vi "Write Idle read.vi"(8 "error in (no error)":errorcluster, 10 "Idle read?":bool, 11 "BaseDriver in":refnum<class "BaseDriver.lvclass">) -> (0 "error out":errorcluster, 3 "BaseDriver out":refnum<class "BaseDriver.lvclass">)   [LabVIEW 2013, in "BaseDriver.lvclass"]
doc: "Determines the drivers behaviour when there is no data to read and no data to send to the remote destination. If Idle Read is true, the driver will wait for data from the remote destination to become available, otherwise it will wait for data from the calling application to become available. It will have slightly faster response time to incoming data from the source it is waiting on.\n\nYour driver should wait for the party that most often initiates communication."
uses:
  BaseDriver.lvclass
  BaseDriver.lvclass/BaseDriver.ctl
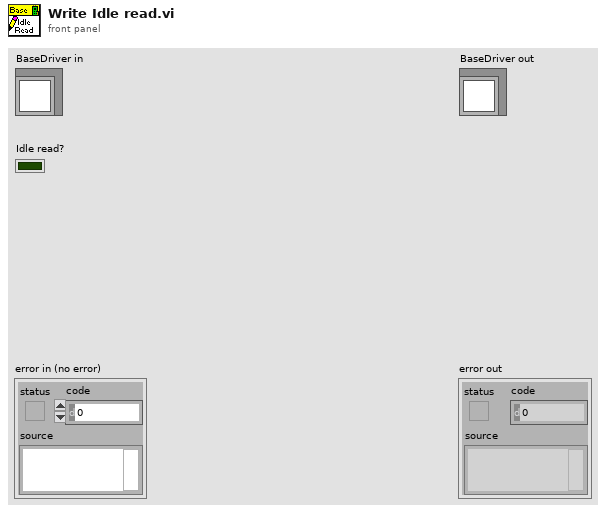
[diagram p1: front panel]
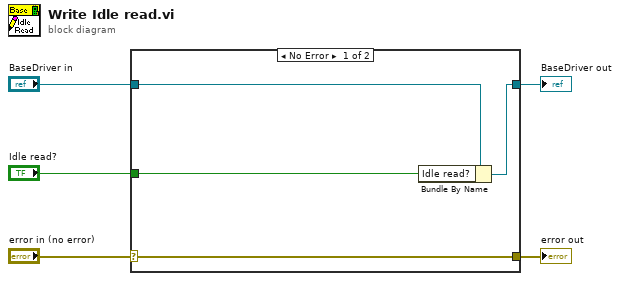
[diagram p0: block diagram]
diagram:
  n1 = case shown="No Error" "error in (no error)" {
    selector: "error in (no error)" -> [w9 w10]
    tunnel: [w9 w10] -> w4
    tunnel: [w7 w11] -> w2
    tunnel: "BaseDriver in" -> [w8 w11]
    tunnel: "Idle read?" -> [w6 _]
    frame No Error {
      n2 = Bundle By Name(cluster=w8, "Idle read?"=w6) -> (w7:refnum<class "BaseDriver.lvclass">)
    }
    frame Error {
    }
  }
  "error out" <- w4
  "BaseDriver out" <- w2
